vi "Find and Rename Classes.vi"(8 "error in (no error)":errorcluster, 10 "New TLB Name":string, 11 "Owned Items[]":refnum<vi>[](array[refnum])) -> (0 "error out":errorcluster, 2 "Array 2":string[](array[string]), 3 "Array":string[](array[string]))   [LabVIEW 2015, in "TLB` Springboard.lvlib"]
uses:
  TLB` Springboard.lvlib
  <vilib>/regexp/Match Regular Expression.xnode
panel:
  in  "Private Data.Application Ref":refnum<vi>
  in  "Private Data.Library Ref":refnum<vi>
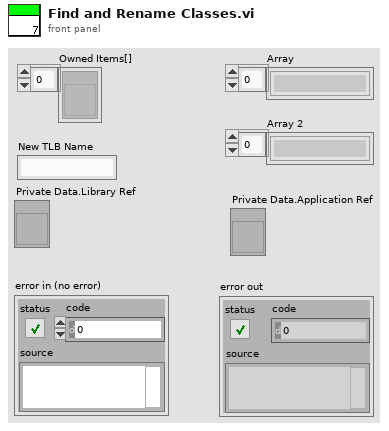
[diagram p1: front panel]
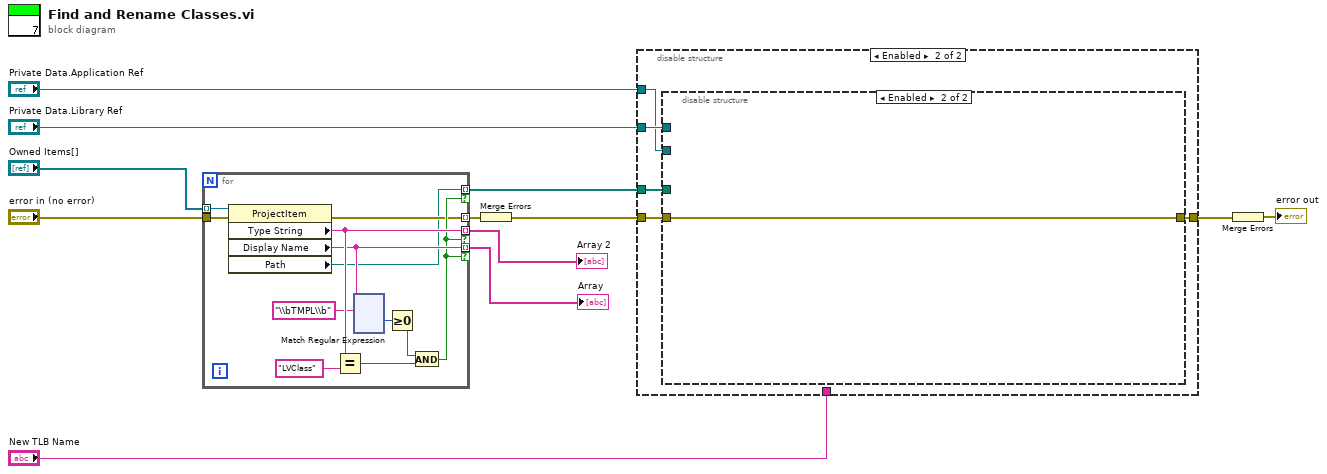
[diagram p0: block diagram]
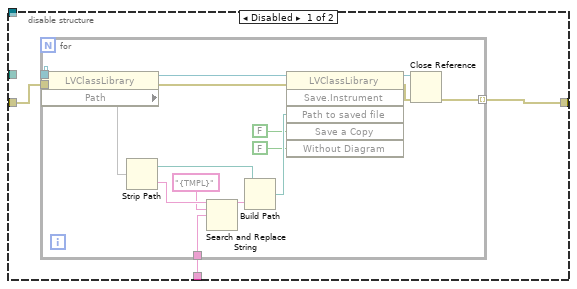
[diagram p2: hidden frame]
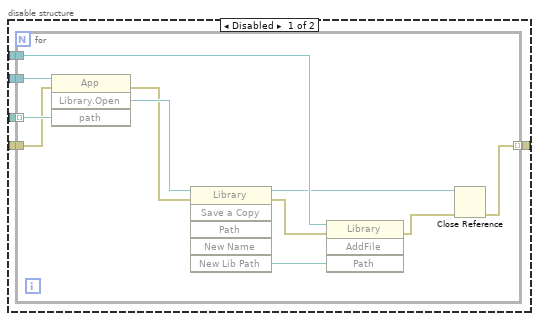
[diagram p3: hidden frame]
diagram:
  n1 = for {
    tunnel: "Owned Items[]" -> [w24] mode=indexing
    tunnel: [w23] -> w7 mode=indexing if=w17
    tunnel: [w20] -> w8 mode=indexing if=w17
    tunnel: [w13] -> w1 mode=indexing if=w17
    tunnel: [w16] -> w11 mode=indexing
    tunnel: "error in (no error)" -> [w15]
    n2 = property class="ProjectItem"(reference=w24, error in=w15) -> (error out=w16:errorcluster, "Type String"=w23:string, "Display Name"=w20:string, "Path"=w13:path)  [unwired: 1 out]
    n3 = Equal?(x=w23, y="LVClass") -> (x = y?=w21:bool)
    n4 = xnode "Match Regular Expression"("input string"=w20, "regular expression"="\\bTMPL\\b") -> ("offset past match"=w18:i32)  [unwired: 4 in, 4 out]
    n5 = Greater Or Equal To 0?(x=w18) -> (x >= 0?=w14:bool)
    n6 = And(x=w14, y=w21) -> (x .and. y?=w17:bool)
  }
  "Array" <- w8
  "Array 2" <- w7
  n7 = Merge Errors(w11) -> (w12:errorcluster)
  n8 = disable-structure shown="Enabled" {
    disable-tunnel: w12 -> [w141 w159]
    disable-tunnel: "New TLB Name" -> [w140 _]
    disable-tunnel: [w139 w158] -> w5
    disable-tunnel: "Private Data.Library Ref" -> [_ w162]
    disable-tunnel: "Private Data.Application Ref" -> [_ w161]
    disable-tunnel: w1 -> [_ w160]
    frame Disabled {
      n9 = for {
        tunnel: w140 -> [w154]
        tunnel: _ -> [w149]
        tunnel: w141 -> [w143]
        tunnel: [w142] -> w139 mode=indexing
        n10 = property class="LVClassLibrary"(reference=w149, error in=w143) -> (reference out=w157:refnum<vi>, error out=w144:errorcluster, "Path"=w156)
        n11 = Strip Path(path=w156) -> (stripped path=w152:path, name=w155:string)
        n12 = Search and Replace String(input string=w155, search string="{TMPL}", replace string=w154) -> (result string=w151:string)  [unwired: 5 in, 3 out]
        n13 = Build Path(base path=w152, name or relative path=w151) -> (appended path=w150:path)
        n14 = invoke class="LVClassLibrary" method="Save.Instrument"(reference=w157, error in=w144, "Path to saved file"=w150, "Save a Copy"=FALSE, "Without Diagram"=FALSE) -> (reference out=w146:refnum<vi>, error out=w145:errorcluster)  [unwired: 1 in, 4 out]
        n15 = Close Reference(reference=w146, error in (no error)=w145) -> (error out=w142:errorcluster)
      }
    }
    frame Enabled {
      n16 = disable-structure shown="Enabled" {
        disable-tunnel: w162 -> [w167 _]
        disable-tunnel: w161 -> [w166 _]
        disable-tunnel: w160 -> [w165 _]
        disable-tunnel: w159 -> [w164 w179]
        disable-tunnel: [w163 w179] -> w158
        frame Disabled {
          n17 = for {
            tunnel: w167 -> [w178]
            tunnel: w166 -> [w177]
            tunnel: w165 -> [w176] mode=indexing
            tunnel: w164 -> [w175]
            tunnel: [w168] -> w163 mode=indexing
            n18 = invoke class="App" method="Library.Open"(reference=w177, error in=w175, "path"=w176) -> (error out=w172:errorcluster, "Open Library"=w174:refnum<vi>)  [unwired: 1 in, 2 out]
            n19 = invoke class="Library" method="Save a Copy"(reference=w174, error in=w172) -> (reference out=w170:refnum<vi>, error out=w171:errorcluster, "New Lib Path"=w173:path)  [unwired: 4 in, 3 out]
            n20 = invoke class="Library" method="AddFile"(reference=w178, error in=w171, "Path"=w173) -> (error out=w169:errorcluster)  [unwired: 1 in, 3 out]
            n21 = Close Reference(reference=w170, error in (no error)=w169) -> (error out=w168:errorcluster)
          }
        }
        frame Enabled {
        }
      }
    }
  }
  n22 = Merge Errors(w5) -> (→"error out":errorcluster)
